vi "curveFit.vi"() -> ()   [LabVIEW 2014]
doc: "This VI reads a spreadsheet .txt data file of theGieger counter and then performs a data decay curve fit with an exponential overlay. This simulated data can also be used to adjust the best guess to fit parameters. The fit reports the lifetime."
uses:
  <vilib>/Utility/file.llb/Read From Spreadsheet File (DBL).vi
panel:
  out "Curve Fit":cluster{"f":dbl[], "y":dbl[]}[](graph)=[{"f"=[0.0, 1.0, 2.0, 3.0, 4.0, 5.0, 6.0, 7.0, 8.0, 9.0, 10.0, 11.0, 12.0, 13.0, 14.0, 15.0, 16.0, 17.0, 18.0, 19.0, 20.0, 21.0, 22.0, 23.0, 24.0, 25.0, 26.0, 27.0, 28.0, 29.0, 30.0, 31.0, 32.0, 33.0, 34.0, 35.0, 36.0, 37.0, 38.0, 39.0, 40.0, 41.0, 42.0, 43.0, 44.0, 45.0, 46.0, 47.0, 48.0, 49.0, 50.0, 51.0, 52.0, 53.0, 54.0, 55.0, 56.0, 57.0, 58.0, 59.0, 60.0, 61.0, 62.0, 63.0, 64.0, 65.0, 66.0, 67.0, 68.0, 69.0, 70.0, 71.0, 72.0, 73.0, 74.0, 75.0, 76.0, 77.0, 78.0, 79.0, 80.0, 81.0, 82.0, 83.0, 84.0, 85.0, 86.0, 87.0, 88.0, 89.0, 90.0, 91.0, 92.0, 93.0, 94.0, 95.0, 96.0, 97.0, 98.0, 99.0, 100.0, 101.0, 102.0, 103.0, 104.0, 105.0, 106.0, 107.0, 108.0, 109.0, 110.0, 111.0, 112.0, 113.0, 114.0, 115.0, 116.0, 117.0, 118.0, 119.0, 120.0, 121.0, 122.0, 123.0, 124.0, 125.0, 126.0, 127.0, 128.0, 129.0, 130.0, 131.0, 132.0, 133.0, 134.0, 135.0, 136.0, 137.0, 138.0, 139.0, 140.0, 141.0, 142.0, 143.0, 144.0, 145.0, 146.0, 147.0, 148.0, 149.0, 150.0, 151.0, 152.0, 153.0, 154.0, 155.0, 156.0, 157.0, 158.0, 159.0, 160.0, 161.0, 162.0, 163.0, 164.0, 165.0, 166.0, 167.0, 168.0, 169.0, 170.0, 171.0, 172.0, 173.0, 174.0, 175.0, 176.0, 177.0, 178.0, 179.0, 180.0, 181.0, 182.0, 183.0, 184.0, 185.0, 186.0, 187.0, 188.0, 189.0, 190.0, 191.0, 192.0, 193.0, 194.0, 195.0, 196.0, 197.0, 198.0, 199.0, 200.0, 201.0, 202.0, 203.0, 204.0, 205.0, 206.0, 207.0, 208.0, 209.0, 210.0, 211.0, 212.0, 213.0, 214.0, 215.0, 216.0, 217.0, 218.0, 219.0, 220.0, 221.0, 222.0, 223.0, 224.0, 225.0, 226.0, 227.0, 228.0, 229.0, 230.0, 231.0, 232.0, 233.0, 234.0, 235.0, 236.0, 237.0, 238.0, 239.0, 240.0, 241.0, 242.0, 243.0, 244.0, 245.0, 246.0, 247.0, 248.0, 249.0, 250.0, 251.0, 252.0, 253.0, 254.0, 255.0, 256.0, 257.0, 258.0, 259.0, 260.0, 261.0, 262.0, 263.0, 264.0, 265.0, 266.0, 267.0, 268.0, 269.0, 270.0, 271.0, 272.0, 273.0, 274.0, 275.0, 276.0, 277.0, 278.0, 279.0, 280.0, 281.0, 282.0, 283.0, 284.0, 285.0, 286.0, 287.0, 288.0, 289.0, 290.0, 291.0, 292.0, 293.0, 294.0, 295.0, 296.0, 297.0, 298.0, 299.0, 300.0], "y"=[0.0, 55.0, 53.0, 56.0, 63.0, 56.0, 61.0, 53.0, 65.0, 65.0, 49.0, 61.0, 63.0, 66.0, 60.0, 56.0, 60.0, 55.0, 54.0, 58.0, 44.0, 50.0, 58.0, 35.0, 47.0, 49.0, 44.0, 53.0, 47.0, 41.0, 62.0, 52.0, 43.0, 50.0, 47.0, 43.0, 47.0, 41.0, 36.0, 37.0, 31.0, 30.0, 44.0, 49.0, 44.0, 38.0, 45.0, 43.0, 42.0, 47.0, 37.0, 35.0, 33.0, 47.0, 42.0, 40.0, 26.0, 36.0, 34.0, 29.0, 37.0, 27.0, 22.0, 26.0, 28.0, 35.0, 32.0, 40.0, 25.0, 26.0, 30.0, 33.0, 25.0, 29.0, 19.0, 26.0, 30.0, 26.0, 27.0, 23.0, 29.0, 22.0, 26.0, 24.0, 24.0, 23.0, 17.0, 24.0, 16.0, 23.0, 25.0, 15.0, 28.0, 28.0, 27.0, 21.0, 21.0, 19.0, 18.0, 17.0, 16.0, 21.0, 22.0, 17.0, 21.0, 14.0, 18.0, 13.0, 14.0, 16.0, 19.0, 19.0, 12.0, 13.0, 27.0, 11.0, 13.0, 18.0, 11.0, 19.0, 18.0, 18.0, 20.0, 13.0, 21.0, 11.0, 19.0, 15.0, 18.0, 20.0, 21.0, 14.0, 19.0, 22.0, 19.0, 13.0, 19.0, 17.0, 9.0, 13.0, 22.0, 16.0, 15.0, 9.0, 17.0, 9.0, 10.0, 12.0, 26.0, 9.0, 15.0, 7.0, 11.0, 14.0, 16.0, 8.0, 10.0, 10.0, 12.0, 12.0, 9.0, 14.0, 11.0, 6.0, 9.0, 11.0, 9.0, 10.0, 12.0, 12.0, 6.0, 10.0, 7.0, 12.0, 12.0, 10.0, 12.0, 16.0, 13.0, 6.0, 12.0, 8.0, 7.0, 7.0, 9.0, 10.0, 13.0, 7.0, 8.0, 4.0, 7.0, 9.0, 9.0, 5.0, 11.0, 8.0, 11.0, 7.0, 9.0, 8.0, 8.0, 8.0, 3.0, 7.0, 9.0, 7.0, 11.0, 7.0, 4.0, 7.0, 6.0, 9.0, 6.0, 7.0, 7.0, 7.0, 5.0, 8.0, 4.0, 10.0, 6.0, 6.0, 9.0, 8.0, 7.0, 6.0, 9.0, 12.0, 7.0, 6.0, 8.0, 3.0, 4.0, 9.0, 9.0, 4.0, 10.0, 6.0, 7.0, 4.0, 2.0, 6.0, 4.0, 4.0, 6.0, 8.0, 6.0, 10.0, 7.0, 6.0, 10.0, 6.0, 6.0, 9.0, 7.0, 3.0, 4.0, 7.0, 10.0, 4.0, 6.0, 6.0, 4.0, 4.0, 5.0, 5.0, 3.0, 7.0, 2.0, 3.0, 6.0, 4.0, 5.0, 4.0, 4.0, 6.0, 5.0, 7.0, 6.0, 3.0, 1.0, 10.0, 5.0, 4.0, 6.0, 8.0, 3.0, 8.0, 4.0, 2.0, 5.0, 3.0, 5.0, 2.0, 0.0, 4.0, 10.0, 3.0, 5.0, 3.0, 3.0]}, {"f"=[0.0, 1.0, 2.0, 3.0, 4.0, 5.0, 6.0, 7.0, 8.0, 9.0, 10.0, 11.0, 12.0, 13.0, 14.0, 15.0, 16.0, 17.0, 18.0, 19.0, 20.0, 21.0, 22.0, 23.0, 24.0, 25.0, 26.0, 27.0, 28.0, 29.0, 30.0, 31.0, 32.0, 33.0, 34.0, 35.0, 36.0, 37.0, 38.0, 39.0, 40.0, 41.0, 42.0, 43.0, 44.0, 45.0, 46.0, 47.0, 48.0, 49.0, 50.0, 51.0, 52.0, 53.0, 54.0, 55.0, 56.0, 57.0, 58.0, 59.0, 60.0, 61.0, 62.0, 63.0, 64.0, 65.0, 66.0, 67.0, 68.0, 69.0, 70.0, 71.0, 72.0, 73.0, 74.0, 75.0, 76.0, 77.0, 78.0, 79.0, 80.0, 81.0, 82.0, 83.0, 84.0, 85.0, 86.0, 87.0, 88.0, 89.0, 90.0, 91.0, 92.0, 93.0, 94.0, 95.0, 96.0, 97.0, 98.0, 99.0, 100.0, 101.0, 102.0, 103.0, 104.0, 105.0, 106.0, 107.0, 108.0, 109.0, 110.0, 111.0, 112.0, 113.0, 114.0, 115.0, 116.0, 117.0, 118.0, 119.0, 120.0, 121.0, 122.0, 123.0, 124.0, 125.0, 126.0, 127.0, 128.0, 129.0, 130.0, 131.0, 132.0, 133.0, 134.0, 135.0, 136.0, 137.0, 138.0, 139.0, 140.0, 141.0, 142.0, 143.0, 144.0, 145.0, 146.0, 147.0, 148.0, 149.0, 150.0, 151.0, 152.0, 153.0, 154.0, 155.0, 156.0, 157.0, 158.0, 159.0, 160.0, 161.0, 162.0, 163.0, 164.0, 165.0, 166.0, 167.0, 168.0, 169.0, 170.0, 171.0, 172.0, 173.0, 174.0, 175.0, 176.0, 177.0, 178.0, 179.0, 180.0, 181.0, 182.0, 183.0, 184.0, 185.0, 186.0, 187.0, 188.0, 189.0, 190.0, 191.0, 192.0, 193.0, 194.0, 195.0, 196.0, 197.0, 198.0, 199.0, 200.0, 201.0, 202.0, 203.0, 204.0, 205.0, 206.0, 207.0, 208.0, 209.0, 210.0, 211.0, 212.0, 213.0, 214.0, 215.0, 216.0, 217.0, 218.0, 219.0, 220.0, 221.0, 222.0, 223.0, 224.0, 225.0, 226.0, 227.0, 228.0, 229.0, 230.0, 231.0, 232.0, 233.0, 234.0, 235.0, 236.0, 237.0, 238.0, 239.0, 240.0, 241.0, 242.0, 243.0, 244.0, 245.0, 246.0, 247.0, 248.0, 249.0, 250.0, 251.0, 252.0, 253.0, 254.0, 255.0, 256.0, 257.0, 258.0, 259.0, 260.0, 261.0, 262.0, 263.0, 264.0, 265.0, 266.0, 267.0, 268.0, 269.0, 270.0, 271.0, 272.0, 273.0, 274.0, 275.0, 276.0, 277.0, 278.0, 279.0, 280.0, 281.0, 282.0, 283.0, 284.0, 285.0, 286.0, 287.0, 288.0, 289.0, 290.0, 291.0, 292.0, 293.0, 294.0, 295.0, 296.0, 297.0, 298.0, 299.0, 300.0], "y"=[60.59549913636967, 59.978638458542484, 59.368057407111195, 58.7636920556349, 58.16547912844226, 57.57335599400671, 56.987260658389076, 56.40713175874694, 55.8329085569101, 55.26453093302141, 54.7019393792424, 54.1450749935229, 53.59387947343415, 53.04829511006469, 52.508264781978326, 51.97373194923366, 51.444640647464524, 50.920935482020575, 50.402561622167674, 49.88946479534715, 49.38159128149368, 48.878887907410835, 48.38130204120403, 47.88878158677004, 47.401274978342705, 46.918731175094074, 46.441099655790545, 45.96833041350343, 45.50037395037335, 45.03718127242787, 44.578703884452025, 44.124893784910896, 43.67570346092402, 43.231085883290866, 42.790994501567, 42.355383239190374, 41.92420648865717, 41.497419106746854, 41.074976409795745, 40.65683416901875, 40.24294860587871, 39.83327638750289, 39.42777462214612, 39.026400854700135, 38.62911306224863, 38.235869649667514, 37.84662944527007, 37.461351696496294, 37.079996065646256, 36.7025226256568, 36.32889185592127, 35.95906463815184, 35.59300225228384, 35.23066637242192, 34.87201906282741, 34.51702277394649, 34.16564033847888, 33.81783496748649, 33.47357024654172, 33.132810131914916, 32.79551894680072, 32.46166137758276, 32.13120247013639, 31.804107626169095, 31.480342599598135, 31.159873492965023, 30.842666753886558, 30.528689171541977, 30.21790787319585, 29.910290320756364, 29.605804307368686, 29.30441795404296, 29.006099706316665, 28.710818330950918, 28.418542912660424, 28.12924285087675, 27.84288785654446, 27.559447948949973, 27.27889345258263, 27.00119499402771, 26.726323498891155, 26.454250188755495, 26.184946578166848, 25.918384471652537, 25.65453596076911, 25.393373421180367, 25.134869509765164, 24.87899716175466, 24.625729587898675, 24.375040271660954, 24.1269029664429, 23.881291692835653, 23.63818073590008, 23.397544642474504, 23.159358218509794, 22.923596526431613, 22.690234882529513, 22.45924885437261, 22.230614258251553, 22.00430715664656, 21.7803038557212, 21.558580902841715, 21.33911508412157, 21.12188342199103, 20.906863172791436, 20.69403182439401, 20.483367093842908, 20.274846925022196, 20.068449486346672, 19.864153168476122, 19.661936582052885, 19.46177855546241, 19.263658132616694, 19.067554570760148, 18.873447338297954, 18.68131611264641, 18.491140778105194, 18.30290142375134, 18.116578341354565, 17.932152023313893, 17.74960316061524, 17.568912640809803, 17.39006154601303, 17.213031150923975, 17.03780292086478, 16.864358509840162, 16.692679758616592, 16.522748692821118, 16.354547521059427, 16.18805863305318, 16.02326459779623, 15.860148161729636, 15.698692246935266, 15.538879949347763, 15.380694536984738, 15.224119448194973, 15.069138289924442, 14.915734836000002, 14.76389302543056, 14.613596960725504, 14.46483090623028, 14.317579286478917, 14.17182668456329, 14.027557840519032, 13.884757649727813, 13.743411161335965, 13.603503576689118, 13.465020247782858, 13.327946675729075, 13.192268509237989, 13.057971543115594, 12.9250417167764, 12.793465112771337, 12.663227955330612, 12.53431660892144, 12.406717576820403, 12.280417499700413, 12.155403154231983, 12.031661451698804, 11.909179436627365, 11.787944285430564, 11.667943305065089, 11.549163931702493, 11.431593729413802, 11.315220388867475, 11.20003172604068, 11.086015680943616, 10.97316031635689, 10.861453816581701, 10.750884486202775, 10.641440748863866, 10.533111146055761, 10.425884335916567, 10.319749092044285, 10.214694302321396, 10.110708967751464, 10.007782201307565, 9.905903226792441, 9.805061377710253, 9.705246096149823, 9.606446931679251, 9.508653540251771, 9.41185568312276, 9.31604322577775, 9.2212061368714, 9.1273344871772, 9.034418448547916, 8.942448292886624, 8.851414391128172, 8.761307212231062, 8.67211732217955, 8.583835382995959, 8.496452151762966, 8.409958479655943, 8.324345310985047, 8.239603682247152, 8.155724721187356, 8.072699645870106, 7.990519763759723, 7.909176470810332, 7.828661250565026, 7.74896567326423, 7.670081394963099, 7.592000156657946, 7.5147137834215325, 7.438214183547185, 7.362493347701594, 7.28754334808627, 7.213356337607512, 7.139924549054837, 7.06724029428778, 6.995295963430947, 6.92408402407729, 6.853597020499475, 6.783827572869293, 6.714768376485, 6.646412201006531, 6.578751889698507, 6.511780358680942, 6.445490596187564, 6.379875661831711, 6.314928685879689, 6.250642868531513, 6.187011479209007, 6.124027855851101, 6.061685404216348, 5.999977597192512, 5.938897974113202, 5.878440140081449, 5.818597765300172, 5.759364584409474, 5.700734395830658, 5.642701061116956, 5.585258504310826, 5.528400711307825, 5.472121729226945, 5.416415665787363, 5.361276688691522, 5.306699025014512, 5.252676960599655, 5.199204839460249, 5.146277063187393, 5.093888090363851, 5.042032435983876, 4.9907046708789435, 4.939899421149334, 4.8896113676014865, 4.839835245191105, 4.790565842471906, 4.741798001050014, 4.69352661504386, 4.64574663054963, 4.598453045112123, 4.551640907201012, 4.505305315692423, 4.459441419355799, 4.414044416345995, 4.369109553700523, 4.324632126841945, 4.2806074790852975, 4.237031001150556, 4.193898130680052, 4.151204351760807, 4.108945194451723, 4.067116234315591, 4.025713091955864, 3.9847314325581413, 3.9441669654363283, 3.904015443583407, 3.864272663226785, 3.8249344633881686, 3.7859967254479265, 3.747455372713866, 3.709306369994423, 3.671545723176181, 3.634169478805705, 3.5971737236756116, 3.5605545844148736, 3.5243082270832846, 3.4884308567700537, 3.452918717196492, 3.4177680903227285, 3.3829752959584494, 3.348536691377584, 3.3144486709369274, 3.280707665698629, 3.2473101430565388, 3.214252606366347, 3.1815315945795017, 3.149143681880835, 3.1170854773298924, 3.0853536245059114, 3.053944801156406, 3.0228557188493435, 2.9920831226288436, 2.9616237906743965, 2.931474533963545, 2.901632195938005, 2.8720936521731737, 2.842855810051013, 2.8139156084362624]}]
  out "Pa Lifetime (s)":dbl=97.73121384022794
  out "Initial Rate (counts/sec)":dbl=60.59549913636967
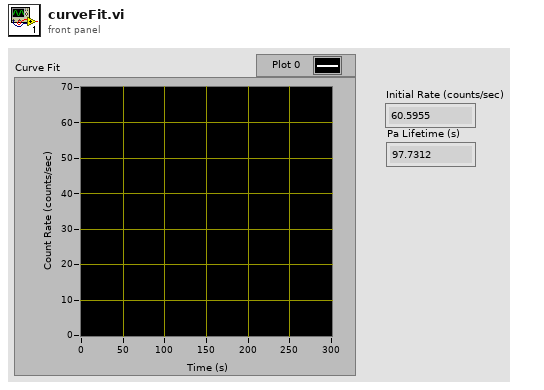
[diagram p1: front panel]
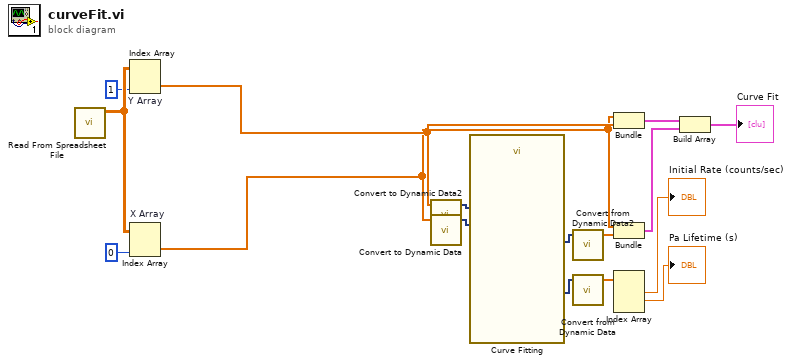
[diagram p0: block diagram]
diagram:
  n1 = call-poly <vilib>:"Read From Spreadsheet File.vi"() -> ("all rows"=w5:dbl[][])  [unwired: 7 in, 4 out]
  n2 = Index Array "Y Array"(array=w5, index (col)=1 ("disabled index (col)")) -> (element=w2:dbl[])  [unwired: 1 in]
  n3 = Index Array "X Array"(array=w5, index (col)=0 ("disabled index (col)")) -> (element=w1:dbl[])  [unwired: 1 in]
  n4 = call "Convert to Dynamic Data2"("Array"=w2) -> ("Dynamic Data Type"=w15:dynamicdata)  [unwired: 3 in]
  n5 = call "Convert to Dynamic Data"("Array"=w1) -> ("Dynamic Data Type"=w16:dynamicdata)  [unwired: 3 in]
  n6 = call "Curve Fitting"("Locations"=w16, "Signals"=w15) -> ("best fit"=w10:dynamicdata, "non-linear coefficients"=w14:dynamicdata)  [unwired: 5 in, 3 out]
  n7 = call "Convert from Dynamic Data2"("Dynamic Data Type"=w10) -> ("Array"=w9:dbl[])  [unwired: 3 in]
  n8 = call "Convert from Dynamic Data"("Dynamic Data Type"=w14) -> ("Array"=w13:dbl[])  [unwired: 3 in]
  n9 = Bundle("all rows"=w1, "all rows"=w2) -> (w7:cluster{"all rows":dbl[], "all rows":dbl[]})  [unwired: 1 in]
  n10 = Bundle("all rows"=w1, "Array"=w9) -> (w8:cluster{"all rows":dbl[], "Array":dbl[]})  [unwired: 1 in]
  n11 = Index Array(array=w13) -> (element #1=→"Initial Rate (counts/sec)":dbl, element #2=→"Pa Lifetime (s)":dbl)  [unwired: 3 in, 1 out]
  n12 = Build Array(w7, w8) -> (→"Curve Fit":cluster{"all rows":dbl[], "Array":dbl[]}[])
